vi "Write Key Value Double.vi"(7 "Section Name":string, 8 "error in (no error)":errorcluster, 9 "Value":dbl, 10 "Key Name":string, 11 "ODBC-Interface in":refnum<class "ODBC-Interface.lvclass">) -> (0 "error out":errorcluster, 2 "found":bool, 3 "ODBC-Interface out":refnum<class "ODBC-Interface.lvclass">)   [LabVIEW 2012, in "DB-Configuration.lvlib" / "ODBC-Interface.lvclass"]
doc: "Write double key value."
uses:
  ODBC-Interface.lvclass
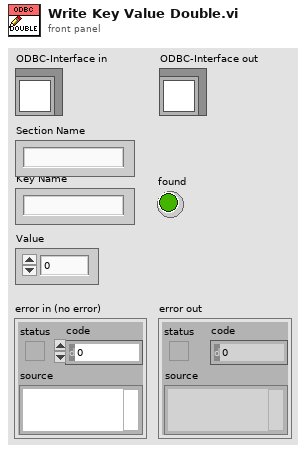
[diagram p1: front panel]
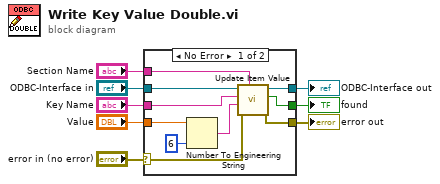
[diagram p0: block diagram]
diagram:
  n1 = case shown="No Error" "error in (no error)" {
    selector: "error in (no error)" -> [w11 w19]
    tunnel: "Section Name" -> [w18 _]
    tunnel: "ODBC-Interface in" -> [w17 w20]
    tunnel: [w16 w20] -> w3
    tunnel: "Key Name" -> [w15 _]
    tunnel: "Value" -> [w10 _]
    tunnel: [w13 w19] -> w1
    tunnel: [w12 _] -> w2
    frame No Error {
      n2 = Number To Engineering String(2:i16 6 ("precision (6)"), 4:w10) -> (0:w14:string)  [unwired: 2 in]
      n3 = call-dynamic "Update Item Value.vi"("Section Name"=w18, "error in (no error)"=w11, "Value"=w14, "Key Name"=w15, "ODBC-Interface in"=w17) -> ("error out"=w13:errorcluster, "found"=w12:bool, "ODBC-Interface out"=w16:refnum<class "ODBC-Interface.lvclass">)  [unwired: 4 in]
    }
    frame Error {
    }
  }
  "error out" <- w1
  "ODBC-Interface out" <- w3
  "found" <- w2
